vi "sec_AlarmColors_main.vi"(7 "Command":T2, 8 "error in (no error)":errorcluster, 10 "Alarm States":T1[](array[typedef]), 11 "Status Zone Refnums":refnum<vi>[](array[refnum])) -> (0 "error out":errorcluster, 3 "Alarm Status":bool[](array[boolean]))   [LabVIEW 2009]
doc: "This Module is responsible for updating the Zone Status Information's color.\nThe color is based on the Alarm State only. \nColors are:\nGreen = Normal\nRed = Alarm\nOrange = Tamper\nBlue = Bypass"
uses:
  sec_AlarmColors_Command_enum.ctl
  controls/sec_AlarmStates_enum.ctl
panel:
  # "Inputs"
  # "Outputs"
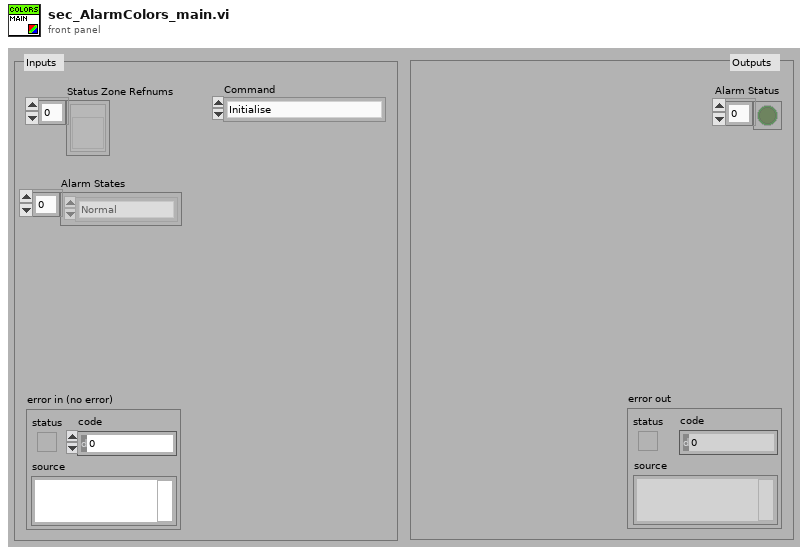
[diagram p1: front panel]
types:
  T1 = typedef "sec_AlarmStates_enum.ctl" = enum16{"Normal", "Alarm", "Bypass", "Tamper"}
  T2 = typedef "sec_AlarmColors_Command_enum.ctl" = enum16{"Initialise", "Set Alarm States", "Update Alarm Status Display", "Shutdown"}
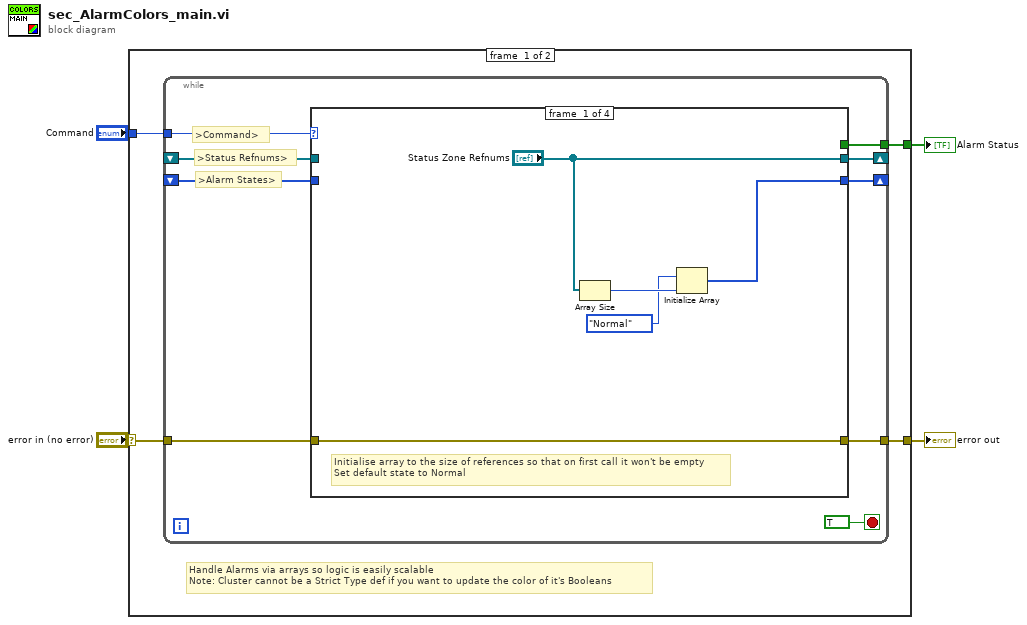
[diagram p0: block diagram]
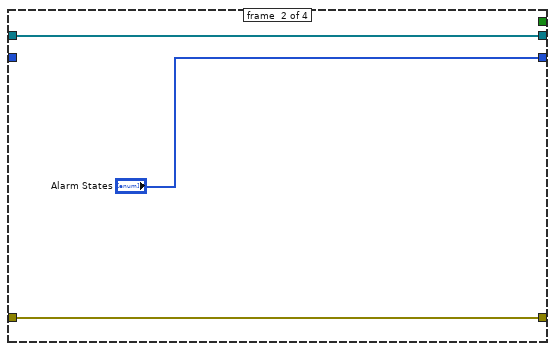
[diagram p2: hidden frame]
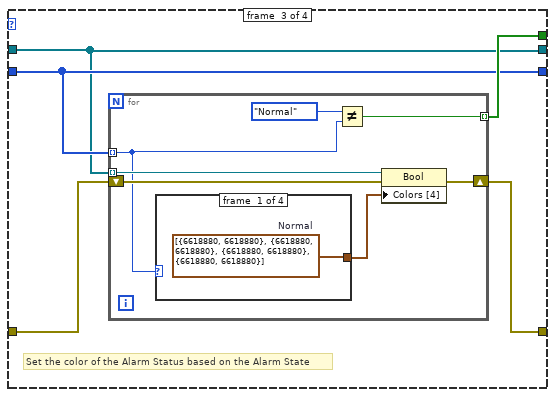
[diagram p3: hidden frame]
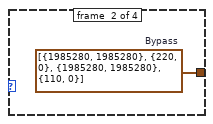
[diagram p4: hidden frame]
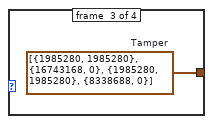
[diagram p5: hidden frame]
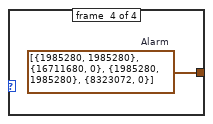
[diagram p6: hidden frame]
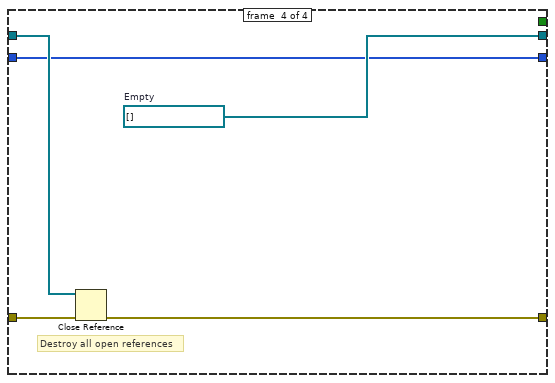
[diagram p7: hidden frame]
diagram:
  n1 = case shown="No Error" "error in (no error)" {
    selector: "error in (no error)" -> [w7 w47]
    tunnel: [w8 w47] -> w3
    tunnel: "Command" -> [w6 _]
    tunnel: [w5 _] -> w1
    frame #0 {
      # "Handle Alarms via arrays so logic is easily scalable\nNote: Cluster cannot be a Strict Type def if you want to update the color of it's Booleans"
      n2 = while {
        tunnel: [w17] -> w8
        tunnel: w7 -> [w16]
        tunnel: w6 -> [w15]
        shift-right: [w14] -> _
        shift-left: _ -> [w13]
        tunnel: [w11] -> w5
        shift-right: [w10] -> _
        shift-left: _ -> [w9]
        stop <- TRUE stop-if-true
        # ">Alarm States>"
        # ">Status Refnums>"
        # ">Command>"
        n3 = case shown="\"Initialise\", Default" w15 {
          tunnel: [w22 w23 w30 w45] -> w17
          tunnel: w16 -> [w22 w23 w29 w46]
          tunnel: ["Status Zone Refnums" w25 w26 w43] -> w14
          tunnel: w13 -> [_ w25 w26 w44]
          tunnel: [_ _ w28 _] -> w11
          tunnel: [w18 "Alarm States" w27 w42] -> w10
          tunnel: w9 -> [_ _ w27 w42]
          frame #0 {
            # "Initialise array to the size of references so that on first call it won't be empty\nSet default state to Normal"
            n4 = Array Size(array="Status Zone Refnums") -> (size(s)=w20:i32)
            n5 = Initialize Array(sec_AlarmStates_enum."Normal" ("Alarm State"), w20) -> (w18:T1[])
          }
          frame #1 {
          }
          frame #2 {
            # "Set the color of the Alarm Status based on the Alarm State"
            n6 = for {
              tunnel: w26 -> [w36] mode=indexing
              shift-right: [w35] -> w30
              shift-left: w29 -> [w37]
              tunnel: [w32] -> w28 mode=indexing
              tunnel: w27 -> [w31] mode=indexing
              n7 = case shown="\"Normal\"" w31 {
                tunnel: [w38 w39 w40 w41] -> w34
                frame #0 {
                  w38 = cluster{u32, u32}[] [{6618880, 6618880}, {6618880, 6618880}, {6618880, 6618880}, {6618880, 6618880}]  # Normal
                }
                frame #1 {
                  w39 = cluster{u32, u32}[] [{1985280, 1985280}, {220, 0}, {1985280, 1985280}, {110, 0}]  # Bypass
                }
                frame #2 {
                  w40 = cluster{u32, u32}[] [{1985280, 1985280}, {16743168, 0}, {1985280, 1985280}, {8338688, 0}]  # Tamper
                }
                frame #3 {
                  w41 = cluster{u32, u32}[] [{1985280, 1985280}, {16711680, 0}, {1985280, 1985280}, {8323072, 0}]  # Alarm
                }
              }
              n8 = Not Equal?(x=sec_AlarmStates_enum."Normal", y=w31) -> (x != y?=w32:bool)
              n9 = property class="Bool"(reference=w36, error in=w37, "Colors [4]"=w34) -> (error out=w35:errorcluster)  [unwired: 1 out]
            }
          }
          frame #3 {
            w43 = refnum<vi>[] []  # Empty
            # "Destroy all open references"
            n10 = Close Reference(reference=w44, error in (no error)=w46) -> (error out=w45:errorcluster)
          }
        }
      }
    }
    frame #1 {
    }
  }
  "error out" <- w3
  "Alarm Status" <- w1
